vi "SUB_SKIP_RS232_TRASH.vi"(3 "error out 2":errorcluster, 4 "read buffer":string, 5 "duplicate VISA resource name 2":refnum<visa-resource-name>) -> (0 "error out":errorcluster, 1 "String":string, 2 "duplicate VISA resource name":refnum<visa-resource-name>)   [LabVIEW 2011]
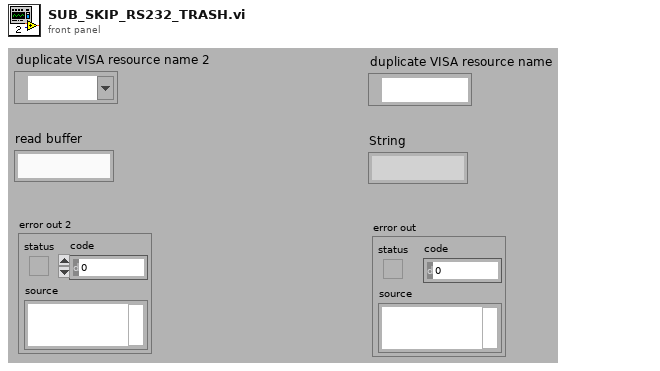
[diagram p1: front panel]
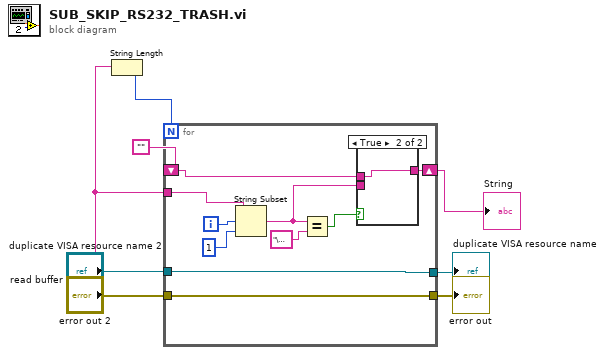
[diagram p0: block diagram]
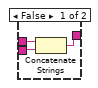
[diagram p2: hidden frame]
diagram:
  n1 = String Length(string="read buffer") -> (length=w1:i32)
  n2 = for {
    N: w1 -> [_]
    shift-right: [w12] -> w4
    shift-left: "" -> [w13]
    tunnel: "read buffer" -> [w11]
    tunnel: "duplicate VISA resource name 2" -> [w10]
    tunnel: [w10] -> w6
    tunnel: [w9] -> w8
    tunnel: "error out 2" -> [w9]
    i -> [w18]
    n3 = String Subset(string=w11, offset (0)=w18, length (rest)=1 ("length (rest)")) -> (substring=w14:string)
    n4 = Equal?(x=w14, y="\u0000") -> (x = y?=w15:bool)
    n5 = case shown="True" w15 {
      tunnel: w14 -> [w21 _]
      tunnel: w13 -> [w20 w22]
      tunnel: [w19 w22] -> w12
      frame False {
        n6 = Concatenate Strings(w20, w21) -> (w19:string)
      }
      frame True {
      }
    }
  }
  "error out" <- w8
  "duplicate VISA resource name" <- w6
  "String" <- w4
